vi "Read_Data_Coils.vi"(8 "error in (no error)":errorcluster, 11 "Device in":refnum<class "MB_TCP_Device.lvclass">) -> (0 "error out":errorcluster, 2 "Discrete Inputs":bool[](array[boolean]), 3 "Device out":refnum<class "MB_TCP_Device.lvclass">)   [LabVIEW 2023, in "MB_TCP_Device.lvclass"]
uses:
  MB_TCP_Device.lvclass
  MB_TCP_Device.lvclass/MB_TCP_Device.ctl
  <vilib>/NI Modbus.llb/MB Ethernet Master Query Read Coils (poly).vi
  <vilib>/numeric/Random Number (Range) I64.vi
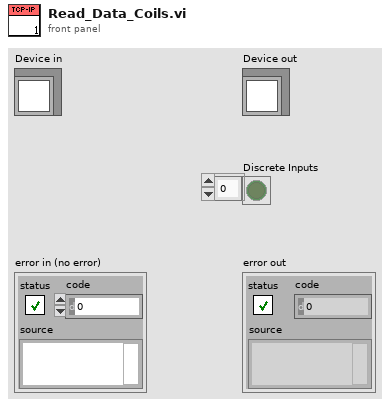
[diagram p1: front panel]
types:
  T1 = typedef "DAQ Device_IO ChannelsData.ctl" = cluster{"#DigitalInputs":u16, "StartAddress_DI":u16, "#DigitalOutputs":u16, "StartAddress_DO":u16, "#AnalogInputs":u16, "StartAddress_AI":u16, "#AnalogOutputs":u16, "StartAddress_AO":u16, "Coil_ReadData":bool[], "Coil_WriteData":bool[], "AI_Data":u16[], "AO_Data":u16[]}
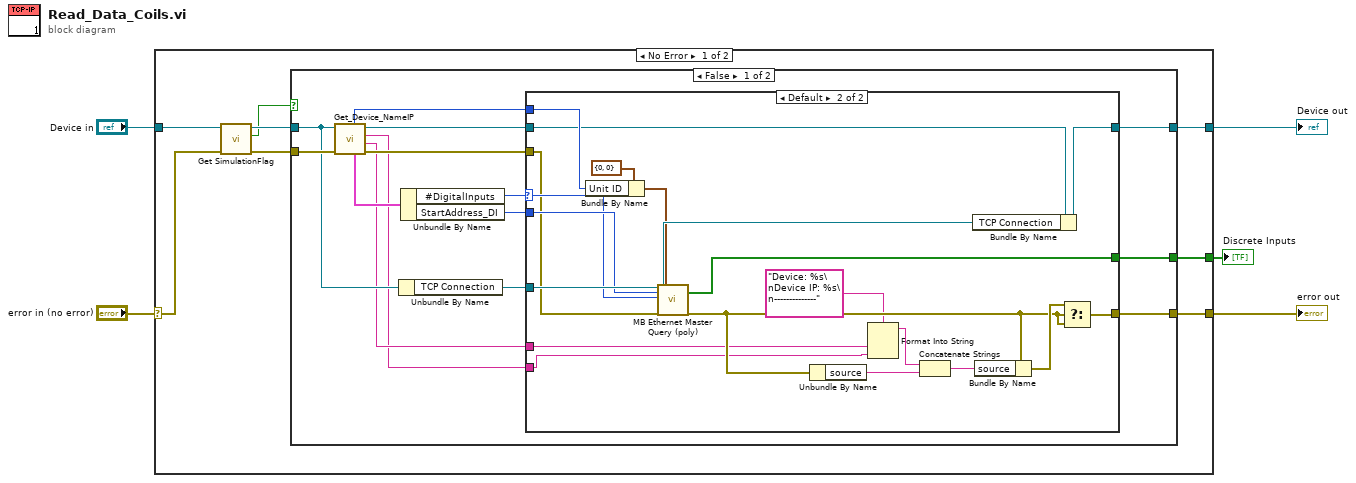
[diagram p0: block diagram]
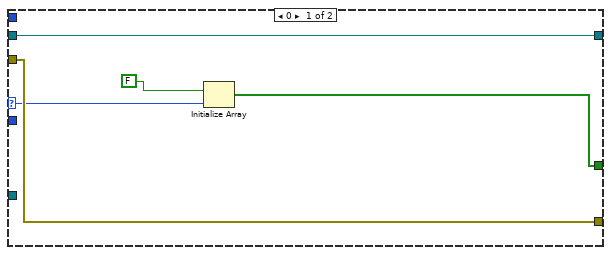
[diagram p2: hidden frame]
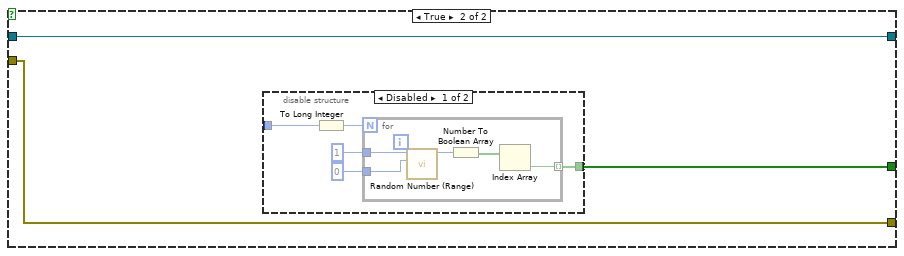
[diagram p3: hidden frame]
diagram:
  n1 = case shown="No Error" "error in (no error)" {
    selector: "error in (no error)" -> [w10 w67]
    tunnel: [w13 w67] -> w4
    tunnel: [w6 w66] -> w2
    tunnel: "Device in" -> [w7 w66]
    tunnel: [w12 _] -> w1
    frame No Error {
      n2 = call-dynamic "Get SimulationFlag.vi"("error in (no error)"=w10, "Device in"=w7) -> ("error out"=w8:errorcluster, "Simulation?"=w9:bool, "Device out"=w11:refnum<class "MB_TCP_Device.lvclass">)  [unwired: 7 in]
      n3 = case shown="False" w9 {
        tunnel: [w27 w54] -> w6
        tunnel: [w26 w53] -> w13
        tunnel: [w25 w55] -> w12
        tunnel: w11 -> [w16 w54]
        tunnel: w8 -> [w22 w53]
        frame False {
          n4 = call-dynamic "Get_Device_NameIP.vi"("error in (no error)"=w22, "Device in"=w16) -> ("error out"=w21:errorcluster, "Device Name"=w15:string, "Device Address"=w14:string, "Device out"=w23:refnum<class "MB_TCP_Device.lvclass">, "IO Channels"=w20:T1, "Unit ID"=w24:u8)  [unwired: 4 in]
          n5 = Unbundle By Name(w16) -> ("TCP Connection"=w17:refnum<k5>)
          n6 = Unbundle By Name(w20) -> ("#DigitalInputs"=w19:u16, "StartAddress_DI"=w18:u16)
          n7 = case shown="Default" w19 {
            selector: w19 -> [w30 w40]
            tunnel: [w32 w52] -> w27
            tunnel: [w31 w48] -> w26
            tunnel: w17 -> [_ w47]
            tunnel: w18 -> [_ w41]
            tunnel: [w28 w42] -> w25
            tunnel: w24 -> [_ w37]
            tunnel: w23 -> [w32 w36]
            tunnel: w21 -> [w31 w35]
            tunnel: w15 -> [_ w34]
            tunnel: w14 -> [_ w33]
            frame 0 {
              n8 = Initialize Array(FALSE, w30) -> (w28:bool[])
            }
            frame Default {
              n9 = Bundle By Name(cluster=cluster{"Transaction ID":u16, "Unit ID":u8} {"Transaction ID"=0, "Unit ID"=0} ("MBAP Header"), "Unit ID"=w37) -> (w38:cluster{"Transaction ID":u16, "Unit ID":u8})
              n10 = call-poly <vilib>:"MB Ethernet Master Query (poly).vi"("TCP Connection Refnum in"=w47, "Starting Address"=w41, "Quantity"=w40, "error in"=w35, "MBAP Header"=w38) -> ("TCP Connection Refnum (dup)"=w51:refnum<k5>, "Coils"=w42:bool[], "error out"=w49:errorcluster)  [unwired: 11 in, 1 out]
              n11 = Unbundle By Name(w49) -> ("source"=w46:string)
              n12 = Format Into String(format string="Device: %s\nDevice IP: %s\n--------------", w34, w33) -> (resulting string=w44:string)  [unwired: 2 in, 1 out]
              n13 = Concatenate Strings(w44, w46) -> (w43:string)
              n14 = Bundle By Name(cluster=w36, "TCP Connection"=w51) -> (w52:refnum<class "MB_TCP_Device.lvclass">)
              n15 = Bundle By Name(cluster=w49, "source"=w43) -> (w50:errorcluster)
              n16 = Select(t=w50, s=w49, f=w49) -> (s? t:f=w48:errorcluster)
            }
          }
        }
        frame True {
          n17 = disable-structure shown="Disabled" {
            disable-tunnel: _ -> [w60 _]
            disable-tunnel: [w56 _] -> w55
            frame Disabled {
              n18 = To Long Integer(number=w60) -> (32bit integer=w59:i32)
              n19 = for {
                N: w59 -> [_]
                tunnel: 1 ("32bit integer") -> [w65]
                tunnel: 0 ("32bit integer") -> [w64]
                tunnel: [w61] -> w56 mode=indexing
                n20 = call-poly <vilib>:"Random Number (Range).vi"("lower bound (-100)"=w64, "upper bound (100)"=w65) -> ("number"=w63:i64)  [unwired: 9 in]
                n21 = Number To Boolean Array(number=w63) -> (Boolean array=w62:bool[])
                n22 = Index Array(array=w62) -> (element=w61:bool)  [unwired: 1 in]
              }
            }
            frame Enabled {
            }
          }
        }
      }
    }
    frame Error {
    }
  }
  "error out" <- w4
  "Device out" <- w2
  "Discrete Inputs" <- w1
